vi "Timing Message Loop.vi"(8 "error in (no error)":errorcluster, 10 "Timers":T1, 11 "Message Queues":T2) -> (0 "error out":errorcluster)   [LabVIEW 2017, in "Message Queue.lvlib"]
uses:
  Message Queue.lvlib
  All Message Queues.ctl
  Message Cluster.ctl
  Acquisition/Acquisition State.ctl
  11995cb8-e311-3fce-f8c0-29dfdff9c03f.vi
  Enqueue Message (Single).vi
  <vilib>/Utility/error.llb/Error Cluster From Error Code.vi
  <vilib>/ErrorRing/Error Ring.xnode
  Acquisition/Acquisition.lvlib
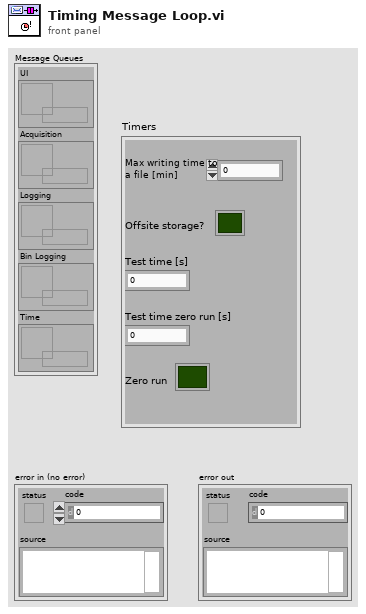
[diagram p1: front panel]
types:
  T1 = cluster{"Offsite storage?":bool, "Test time [s]":dbl, "Test time zero run [s] ":dbl, "Max writing time to a file [min]":dbl, "Zero run":bool}
  T2 = typedef "Message Queue.lvlib/All Message Queues.ctl" = cluster{"UI":refnum<queue>, "Acquisition":refnum<queue>, "Logging":refnum<queue>, "Bin Logging":refnum<queue>, "Time":refnum<queue>}
  T3 = typedef "Acquisition.lvlib/Acquisition State.ctl" = enum16{"Idle", "Acquiring"}
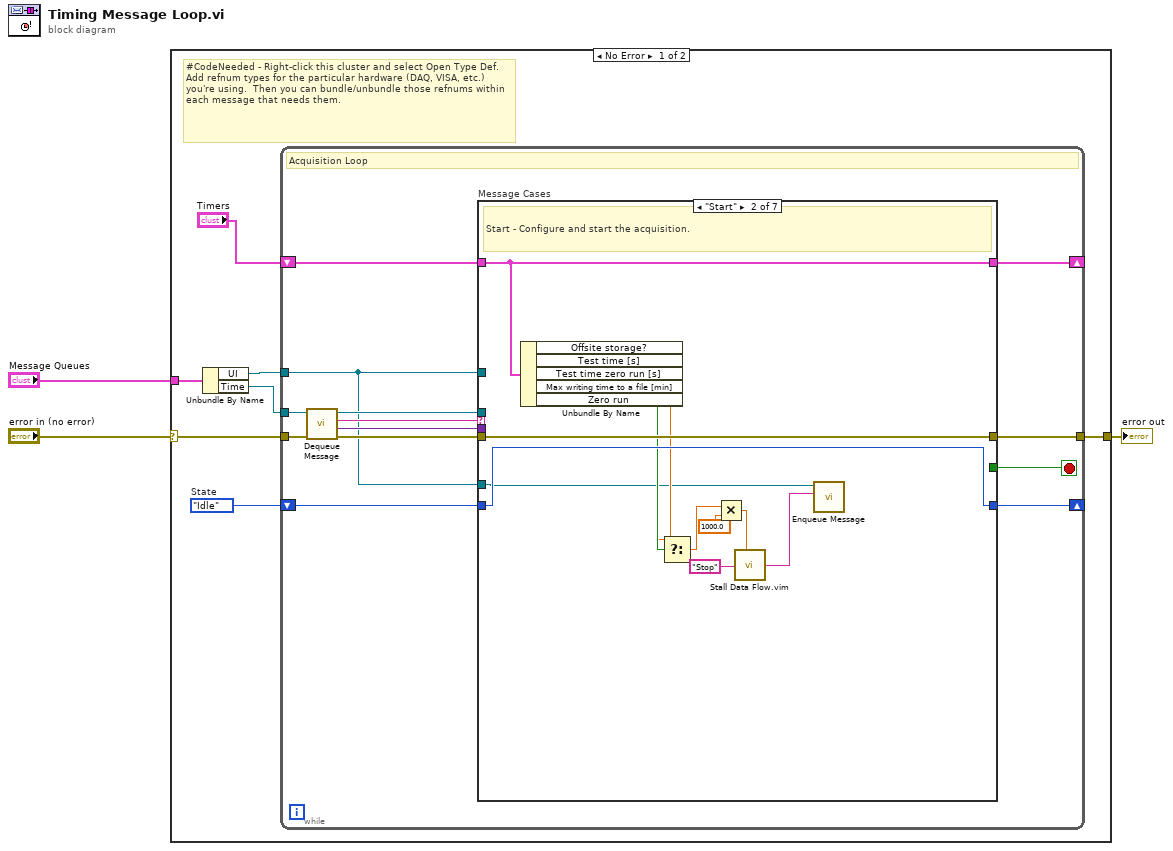
[diagram p0: block diagram]
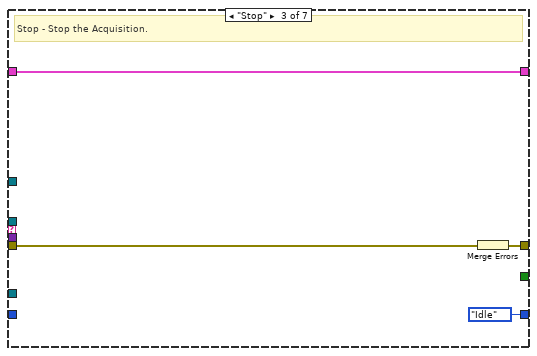
[diagram p3: hidden frame]
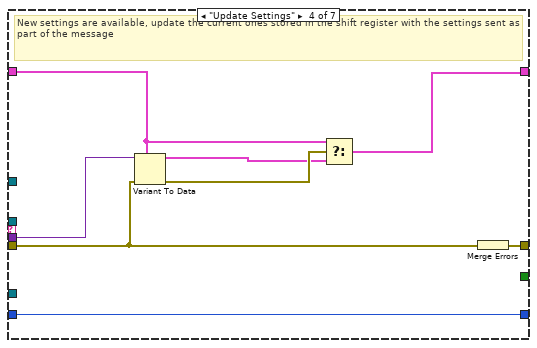
[diagram p4: hidden frame]
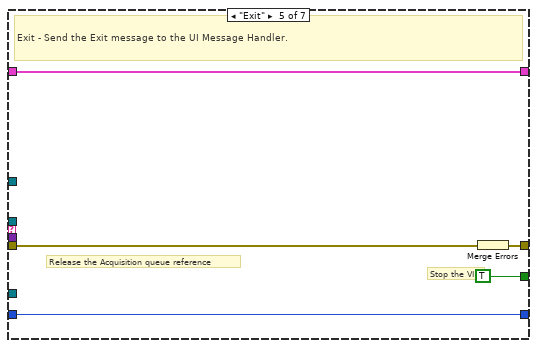
[diagram p5: hidden frame]
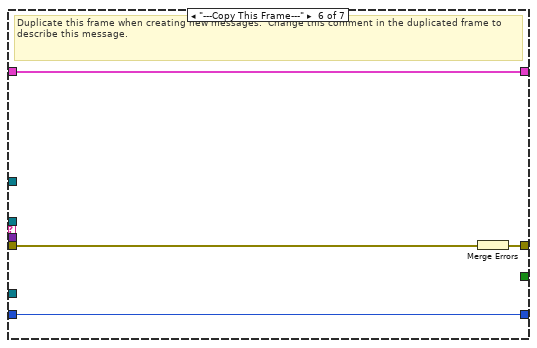
[diagram p6: hidden frame]
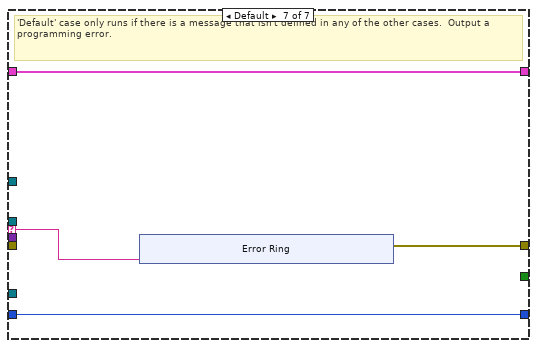
[diagram p7: hidden frame]
diagram:
  n1 = case shown="No Error" "error in (no error)" {
    selector: "error in (no error)" -> [w8 w71]
    tunnel: "Message Queues" -> [w10 _]
    tunnel: [w4 w71] -> w2
    frame No Error {
      w6 = Acquisition_State."Idle"  # State
      # "#CodeNeeded - Right-click this cluster and select Open Type Def.  Add refnum types for the particular hardware (DAQ, VISA, etc.) you're using.  Then you can bundle/unbundle those refnums within each message that needs them."
      n2 = Unbundle By Name(w10) -> ("UI"=w7:refnum<queue>, "Time"=w9:refnum<queue>)
      n3 = while {
        tunnel: w9 -> [w16]
        shift-right: [w22] -> _
        shift-left: "Timers" -> [w23]
        tunnel: w7 -> [w12]
        shift-right: [w14] -> _
        shift-left: w6 -> [w15]
        tunnel: w8 -> [w20]
        tunnel: [w11] -> w4
        stop <- w21 stop-if-true
        # "Acquisition Loop"
        n4 = call "Dequeue Message.vi"("error in (no error)"=w20, "Message Queue"=w16) -> ("error out"=w19:errorcluster, "Message Data"=w17:variant, "Message"=w18:string, "dup Message Queue"=w13:refnum<queue>)  [unwired: 6 in]
        n5 = case "Message Cases" shown="\"Start\"" w18 {
          selector: w18 -> [_ _ _ _ _ _ w60]
          tunnel: w13 -> [_ _ _ _ _ _ _]
          tunnel: w19 -> [w26 w38 w40 w46 w51 w59 _]
          tunnel: [w26 w38 w42 w50 w54 w57 w61] -> w11
          tunnel: w23 -> [w25 w31 w41 w43 w53 w58 w63]
          tunnel: [w25 w31 w41 w47 w53 w58 w63] -> w22
          tunnel: [_ _ _ _ TRUE _ _] -> w21
          tunnel: w17 -> [_ _ _ w44 _ _ _]
          tunnel: w12 -> [_ _ _ _ _ _ _]
          tunnel: w15 -> [w24 w37 _ w45 w52 w56 w62]
          tunnel: [w24 w37 Acquisition_State."Idle" ("State") w45 w52 w56 w62] -> w14
          tunnel: w12 -> [_ w27 _ _ _ _ _]
          frame "Initialize" {
            # "Initialize  - Initialize is currently a no-op.  The hardware initialization takes place in the 'Start' message."
          }
          frame "Start" {
            # "Start - Configure and start the acquisition."
            n6 = Unbundle By Name(w31) -> ("Test time [s]"=w34:dbl, "Test time zero run [s]"=w33:dbl, "Zero run"=w35:bool)  [unwired: 2 out]
            n7 = Select(t=w33, s=w35, f=w34) -> (s? t:f=w32:dbl)
            n8 = Multiply(x=w32, y=1000.0) -> (x*y=w30:dbl)
            n9 = call "Stall Data Flow.vim"("value in"="Stop" ("Message"), "milliseconds to wait"=w30) -> ("value out"=w28:string)  [unwired: 1 out]
            n10 = call-poly "Enqueue Message.vi"("Message"=w28, "Message Queue"=w27) -> ()  [unwired: 8 in, 2 out]
          }
          frame "Stop" {
            # "Stop - Stop the Acquisition."
            n11 = Merge Errors(w40) -> (w42:errorcluster)
          }
          frame "Update Settings" {
            # "New settings are available, update the current ones stored in the shift register with the settings sent as part of the message"
            n12 = Variant To Data(error in=w46, type=w43, Variant=w44) -> (data=w48:T1, error out=w49:errorcluster)
            n13 = Select(t=w43, s=w49, f=w48) -> (s? t:f=w47:T1)
            n14 = Merge Errors(w46) -> (w50:errorcluster)
          }
          frame "Exit" {
            # "Release the Acquisition queue reference"
            # "Stop the VI"
            # "Exit - Send the Exit message to the UI Message Handler."
            n15 = Merge Errors(w51) -> (w54:errorcluster)
          }
          frame "---Copy This Frame---" {
            # "Duplicate this frame when creating new messages.  Change this comment in the duplicated frame to describe this message."
            n16 = Merge Errors(w59) -> (w57:errorcluster)
          }
          frame Default {
            # "'Default' case only runs if there is a message that isn't defined in any of the other cases.  Output a programming error."
            n17 = xnode "Error Ring"("parameter 0"=w60) -> ("error out"=w61:errorcluster)
          }
        }
      }
    }
    frame Error {
    }
  }
  "error out" <- w2
